vi "Wristband main - Pinch Leap based2.vi"() -> ()   [LabVIEW 2014]
uses:
  Typedef/sensor_data.ctl
  Typedef/flexext_data.ctl
  Typedef/pinch_data.ctl
  SubVIs/Save Blocks - 2D.vi
  <vilib>/MakerHub/LINX/Public/Peripherals/Analog/Analog Read N Chans.vi
  <vilib>/MakerHub/LINX/LMH-LINX.lvlib
panel:
  out "Pinch cluster":T1
  in  "X Scale.Range:Maximum":dbl=200.0 format="%#_13g"
  in  "X Scale.Range:Minimum":dbl format="%#_13g"
  in  "X-scale change":bool
  in  "Clear Plot":bool
  in  "Acquire":bool
  in  "Tacq":u32=50 caption="Acquisition Interval" min=50 max=10000 step=50 format="%.0fms"
  in  "N pts":i32=500
  in  "Session name":string="Sessione Mat"
  in  "Save to path":path=path "C:/Users/Arquilla/Documents/Matteo/Documents/Matteo/Università/Campus Biomedico/Tesi Magistrale/smart wrist save"
  out "Leap \nConnected?":bool=TRUE caption="Leap Motion"
  in  "Arduino Port":refnum<visa-resource-name>
  out "Status":bool caption="Arduino"
  out "Sensor Chart":T2(graph)
  out "Grab Strength":u8
  out "Flexext cluster":T3
  out "Sensor Data":T4={"Sensor  Chan 0"=1.66015625, "Sensor Chan 1"=2.060546875, "Sensor Chan 2"=2.099609375, "Sensor Chan 3"=2.12890625, "Sensor Chan 4"=2.0751953125, "Sensor Chan 5"=1.8115234375}
  in  "Exit":bool
  out "Event Chart":T5(graph)
  # "Connection panel"
  # "Acquisition panel"
  # "Save settings"
  # "Connection status"
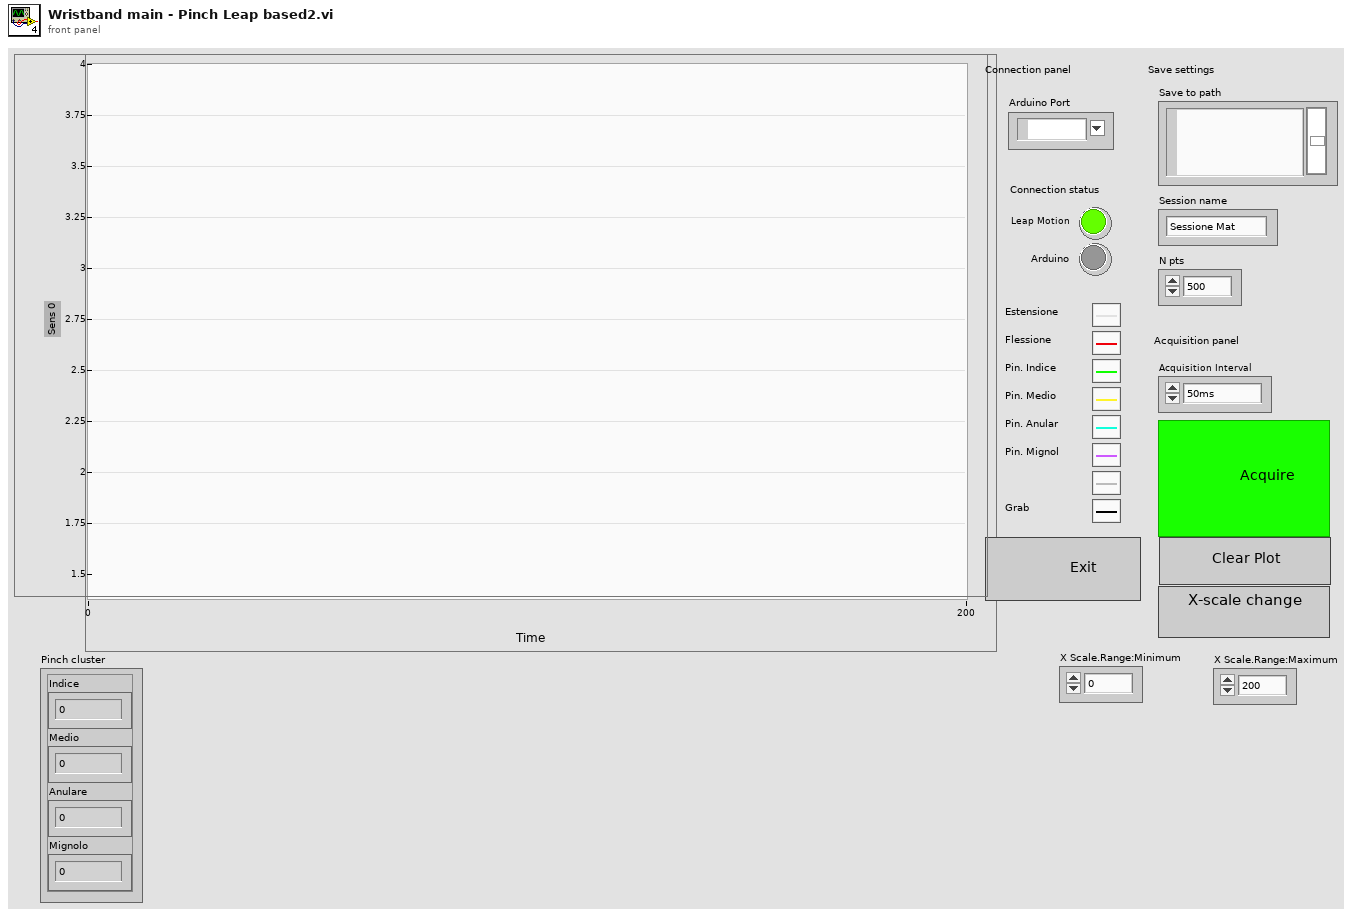
[diagram p1: front panel]
types:
  T1 = typedef "pinch_data.ctl" = cluster{"Indice":u8, "Medio":u8, "Anulare":u8, "Mignolo":u8}
  T2 = cluster{"Sensor  Chan 0":dbl, "Sensor Chan 2":dbl, "Sensor Chan 4":dbl, "Sensor Chan 5":dbl}
  T3 = typedef "flexext_data.ctl" = cluster{"Estensione":u8, "Flessione":u8}
  T4 = typedef "Sensor_data.ctl" = cluster{"Sensor  Chan 0":dbl, "Sensor Chan 1":dbl, "Sensor Chan 2":dbl, "Sensor Chan 3":dbl, "Sensor Chan 4":dbl, "Sensor Chan 5":dbl}
  T5 = cluster{"Estensione":u8, "Flessione":u8, "Indice":u8, "Medio":u8, "Anulare":u8, "Mignolo":u8, "Grab Strength":u8}
  T6 = typedef "LMH-LINX.lvlib/LINX Ref.ctl" = cluster{"Platform":T7, "Interface":T8, "LINX Device Config":T9}
  T7 = typedef "LMH-LINX.lvlib/Platform.ctl" = enum16{"LINX", "myRIO"}
  T8 = typedef "LMH-LINX.lvlib/Interface.ctl" = enum16{"Serial", "TCP"}
  T9 = typedef "LMH-LINX.lvlib/Device.lvlib/LINX Device Config.ctl" = cluster{"Interface":T8, "COM Port":refnum<visa-resource-name>, "TCP Configuration":T10, "Device Family":u8, "Device ID":u8, "Device Name":string, "TCP Ref":refnum<k5>, "Channels":T11}
  T10 = typedef "LMH-LINX.lvlib/Device.lvlib/TCP Config.ctl" = cluster{"IP Address":string, "Port":u16}
  T11 = typedef "LMH-LINX.lvlib/Channels.ctl" = cluster{"DI":u8[], "DO":u8[], "AI":u8[], "AO":u8[], "PWM":u8[], "QE":u8[], "UART":u8[], "I2C 2":u8[], "SPI":u8[], "CAN":u8[], "Servo":u8[], "AI Ref (V)":dbl, "AO Ref (V)":dbl, "AO Resolution (Bits)":u8}
  T12 = typedef "Leap Handle.ctl" = cluster{"LeapCSharp":refnum<k24>}
  T13 = cluster{"Estensione":u8, "Flessione":u8, "Indice":u8, "Medio":u8, "Anulare":u8, "Mignolo":u8, "Grab Strength":u8}[]
  T14 = cluster{"Sensor  Chan 0":dbl, "Sensor Chan 2":dbl, "Sensor Chan 4":dbl, "Sensor Chan 5":dbl}[]
  T15 = cluster{"Sensor  Chan 0":dbl, "Sensor Chan 1":dbl, "Sensor Chan 2":dbl, "Sensor Chan 3":dbl}
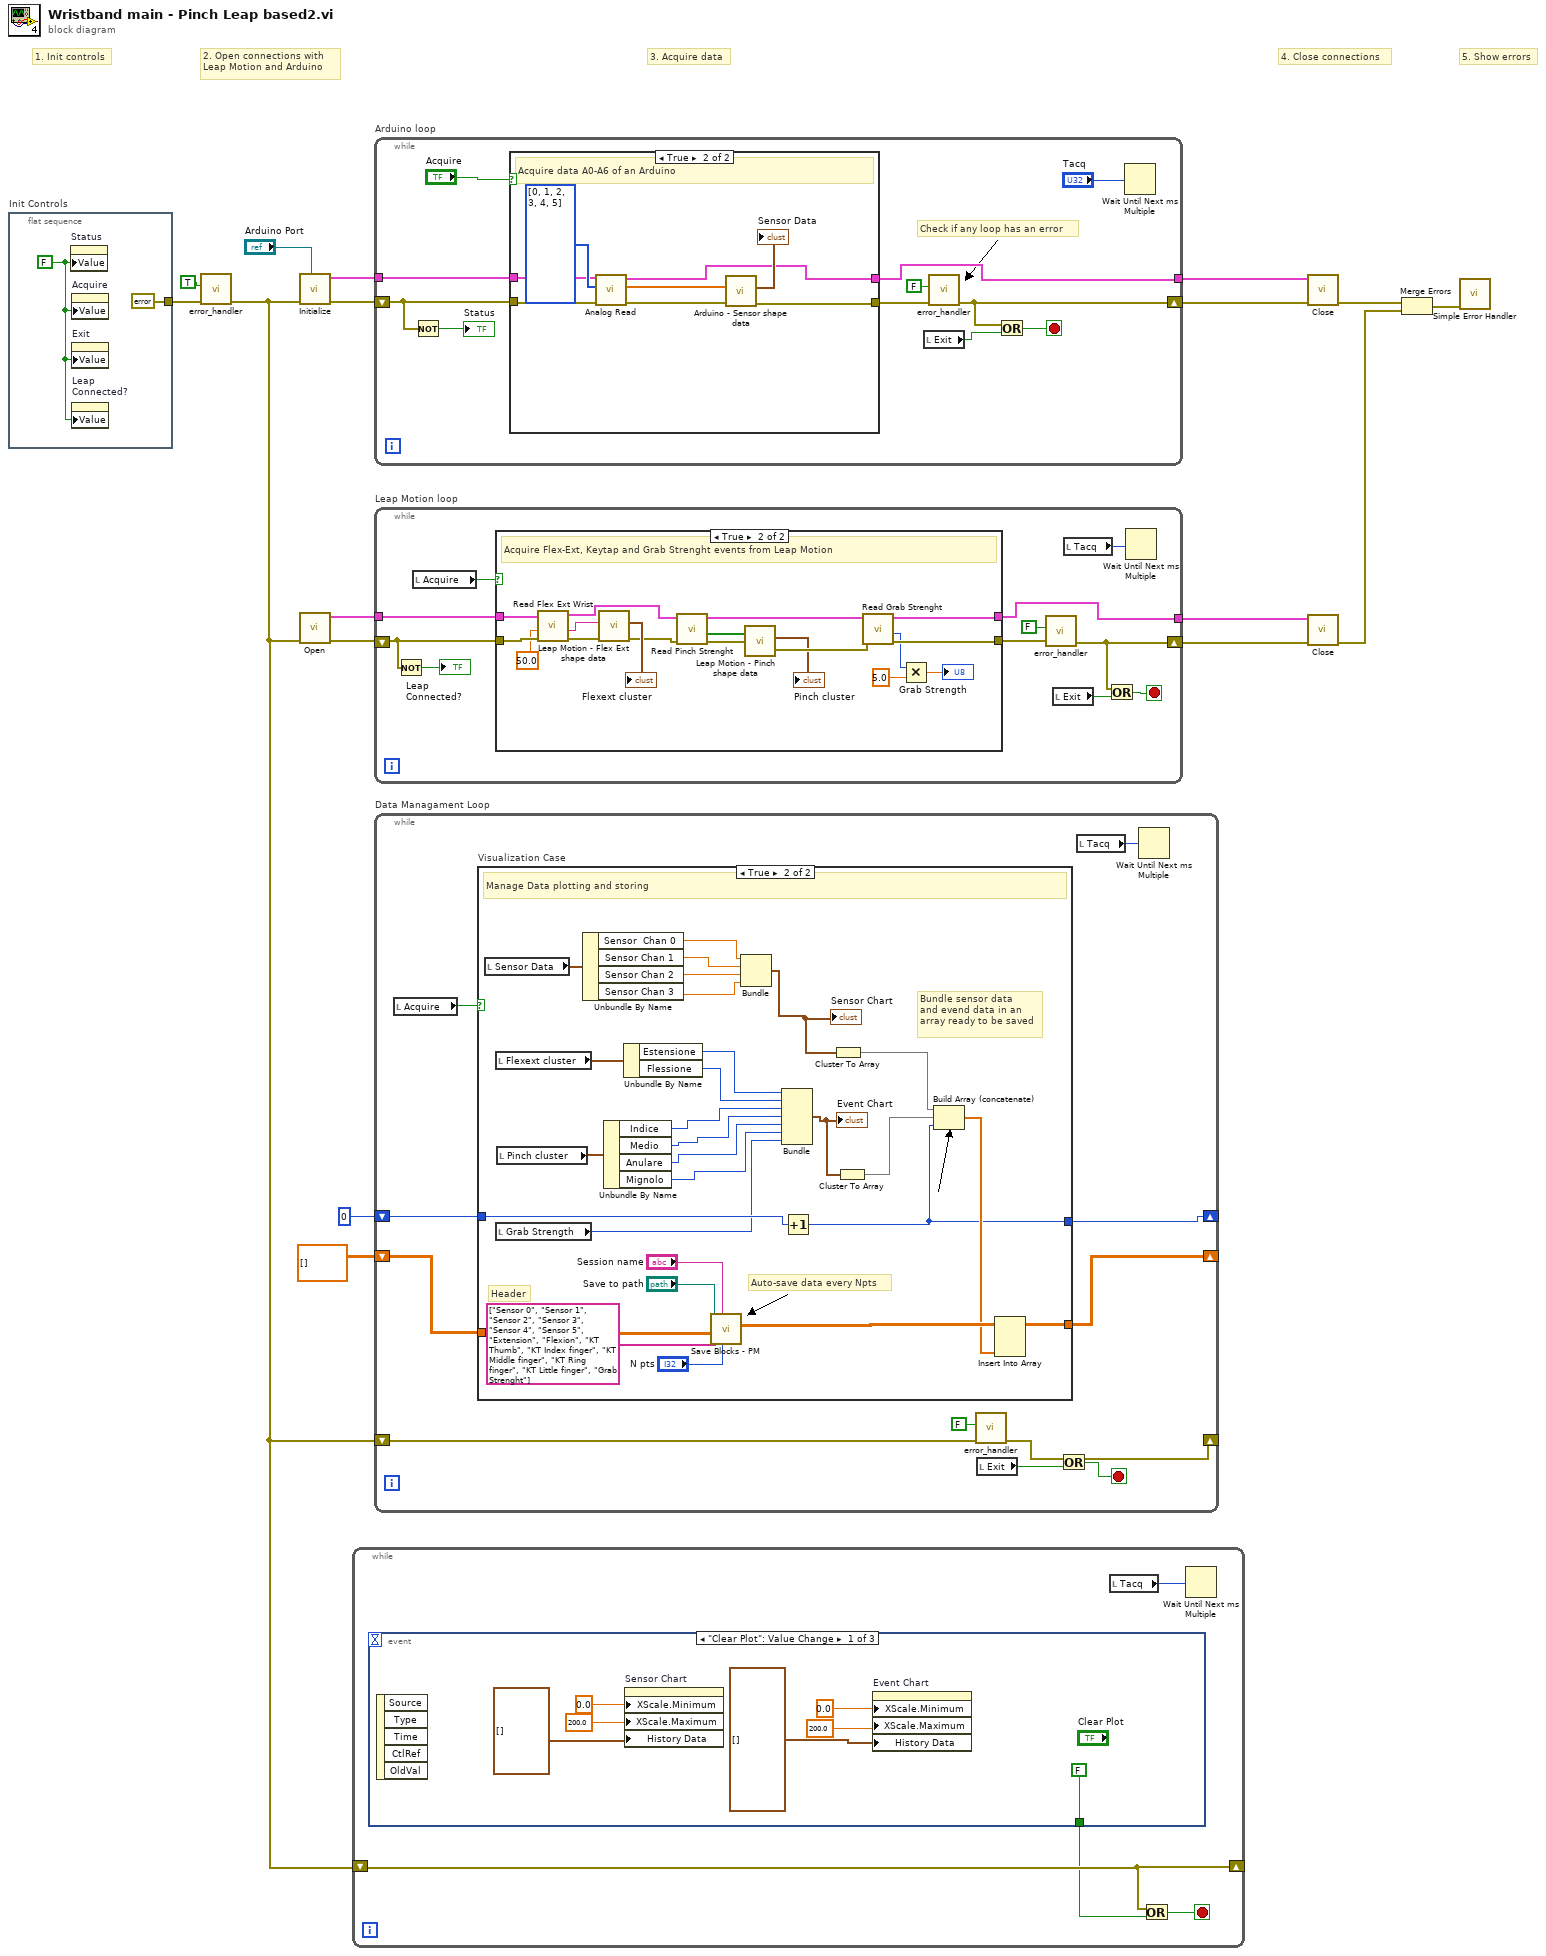
[diagram p0: block diagram]
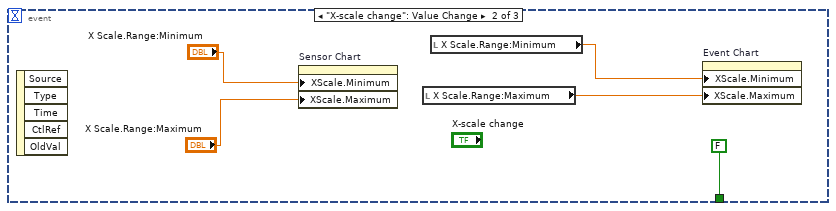
[diagram p2: hidden frame]
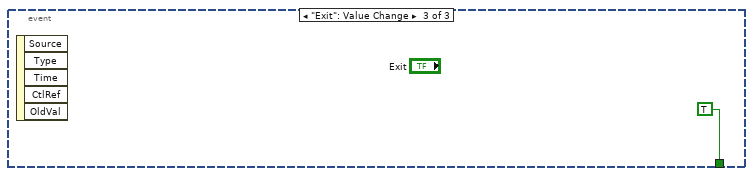
[diagram p3: hidden frame]
diagram:
  # "5. Show errors"
  # "4. Close connections"
  # "3. Acquire data"
  # "2. Open connections with\nLeap Motion and Arduino"
  # "1. Init controls"
  n1 = flat-sequence "Init Controls" {
    tunnel: [errorcluster {"status"=FALSE, "code"=0, "source"=""} ("Error In")] -> w8
    frame #0 {
      w18 = FALSE ("Status")
      n2 = property on="Status" class="Bool (strict)"("Value"=w18) -> ()  [unwired: 2 in, 2 out]
      n3 = property on="Acquire" class="Bool (strict)"("Value"=w18) -> ()  [unwired: 2 in, 2 out]
      n4 = property on="Exit" class="Bool (strict)"("Value"=w18) -> ()  [unwired: 2 in, 2 out]
      n5 = property on="Leap \nConnected?" class="Bool (strict)"("Value"=w18) -> ()  [unwired: 2 in, 2 out]
    }
  }
  n6 = call "error_handler.vi"("Error In"=w8, "Reset"=TRUE) -> ("Error Out"=w2:errorcluster)  [unwired: 9 in]
  n7 = call <vilib>:"Initialize.vi"("Serial Port"="Arduino Port", "Error In"=w2) -> ("Error Out"=w16:errorcluster, "LINX Ref"=w17:T6)  [unwired: 7 in, 1 out]
  n8 = call "Open.vi"("Error In"=w2) -> ("Error Out"=w11:errorcluster, "Leap Handle"=w12:T12)  [unwired: 9 in]
  n9 = while {
    shift-right: [w21] -> _
    shift-left: w2 -> [w21]
    stop <- w22 stop-if-true
    n10 = event shown="[0] \"Clear Plot\": Value Change" {
      selector: _ -> [_ _ _]
      dyn-events: _ -> [_ _ _]
      timeout: _ -> [_ _ _]
      tunnel: [FALSE FALSE TRUE] -> w20
      event "Clear Plot": Value Change {
        n11 = event-data() -> ()  [unwired: 1 in, 5 out]
        n12 = property on="Sensor Chart" class="WFChart (strict)"("XScale.Minimum"=0.0 ("X Scale.Range:Minimum"), "XScale.Maximum"=200.0 ("X Scale.Range:Maximum"), "History Data"=T14 []) -> ()  [unwired: 2 in, 2 out]
        n13 = property on="Event Chart" class="WFChart (strict)"("XScale.Minimum"=0.0 ("X Scale.Range:Minimum"), "XScale.Maximum"=200.0 ("X Scale.Range:Maximum"), "History Data"=T13 []) -> ()  [unwired: 2 in, 2 out]
      }
      event "X-scale change": Value Change {
        n14 = event-data() -> ()  [unwired: 1 in, 5 out]
        n15 = property on="Sensor Chart" class="WFChart (strict)"("XScale.Minimum"="X Scale.Range:Minimum", "XScale.Maximum"="X Scale.Range:Maximum") -> ()  [unwired: 2 in, 2 out]
        n16 = local read "X Scale.Range:Maximum"() -> (w31:dbl)
        n17 = local read "X Scale.Range:Minimum"() -> (w34:dbl)
        n18 = property on="Event Chart" class="WFChart (strict)"("XScale.Minimum"=w34, "XScale.Maximum"=w31) -> ()  [unwired: 2 in, 2 out]
      }
      event "Exit": Value Change {
        n19 = event-data() -> ()  [unwired: 1 in, 5 out]
      }
    }
    n20 = local read "Tacq"() -> (w23:u32)
    n21 = Or(x=w21, y=w20) -> (x .or. y?=w22:bool)
    n22 = Wait Until Next ms Multiple(millisecond multiple=w23) -> ()  [unwired: 1 out]
  }
  n23 = while "Arduino loop" {
    tunnel: w17 -> [w46]
    tunnel: [w39] -> w13
    shift-right: [w40] -> w14
    shift-left: w16 -> [w43]
    stop <- w45 stop-if-true
    # "Check if any loop has an error"
    n24 = Not(x=w43) -> (.not. x?=→"Status":bool)
    n25 = case shown="True" "Acquire" {
      tunnel: w46 -> [w48 w55]
      tunnel: w43 -> [w49 w57]
      tunnel: [w48 w50] -> w39
      tunnel: [w49 w53] -> w41
      frame False {
        # "Idle"
      }
      frame True {
        # "Acquire data A0-A6 of an Arduino"
        n26 = call-poly <vilib>:"Analog Read.vi"("Error In"=w57, "AI Channel(s)"=u8[] [0, 1, 2, 3, 4, 5], "LINX Resource"=w55) -> ("Error Out"=w54:errorcluster, "Voltages"=w52:dbl[], "LINX Resource"=w50:T6)  [unwired: 5 in, 1 out]
        n27 = call "Arduino - Sensor shape data.vi"("Error In"=w54, "Sensor Data in"=w52) -> ("Error Out"=w53:errorcluster, "Sensor Data Out"=→"Sensor Data":T4)  [unwired: 8 in]
      }
    }
    n28 = local read "Exit"() -> (w37:bool)
    n29 = call "error_handler.vi"("Error In"=w41, "Reset"=FALSE) -> ("Error Out"=w40:errorcluster)  [unwired: 9 in]
    n30 = Or(x=w40, y=w37) -> (x .or. y?=w45:bool)
    n31 = Wait Until Next ms Multiple(millisecond multiple="Tacq") -> ()  [unwired: 1 out]
  }
  n32 = while "Leap Motion loop" {
    tunnel: w12 -> [w66]
    tunnel: [w60] -> w10
    shift-right: [w62] -> w9
    shift-left: w11 -> [w59]
    stop <- w67 stop-if-true
    n33 = Not(x=w59) -> (.not. x?=→"Leap \nConnected?":bool)
    n34 = local read "Acquire"() -> (w64:bool)
    n35 = case shown="True" w64 {
      tunnel: w66 -> [w70 w88]
      tunnel: w59 -> [w69 w87]
      tunnel: [w70 w82] -> w60
      tunnel: [w69 w81] -> w63
      frame False {
        # "Idle"
      }
      frame True {
        # "Acquire Flex-Ext, Keytap and Grab Strenght events from Leap Motion"
        n36 = call "Read Flex Ext Wrist.vi"("Error In"=w87, "Flex Extension threshold"=sgl 50.0, "Leap Handle In"=w88) -> ("Error Out"=w85:errorcluster, "Wrist Flextion/Extension"=w84:string, "Leap Handle Out"=w77:T12)  [unwired: 4 in]
        n37 = call "Leap Motion - Flex Ext shape data.vi"("Error In"=w85, "Event In"=w84) -> ("Error Out"=w76:errorcluster, "Flexext cluster"=→"Flexext cluster":T3)  [unwired: 8 in]
        n38 = call "Read Pinch Strenght.vi"("Error In"=w76, "Leap Handle In"=w77) -> ("Error Out"=w74:errorcluster, "Finger pinch"=w73:bool[], "Leap Handle Out"=w75:T12)  [unwired: 6 in, 1 out]
        n39 = call "Leap Motion - Pinch shape data.vi"("Error In"=w74, "Pinch"=w73) -> ("Error Out"=w72:errorcluster, "Pinch cluster"=→"Pinch cluster":T1)  [unwired: 8 in]
        n40 = call "Read Grab Strenght.vi"("Error In"=w72, "Leap Handle In"=w75) -> ("Error Out"=w81:errorcluster, "Numeric Palm State"=w78:i32, "Leap Handle Out"=w82:T12)  [unwired: 5 in, 2 out]
        n41 = Multiply(x=w78, y=sgl 5.0) -> (x*y=→"Grab Strength":sgl)
      }
    }
    n42 = call "error_handler.vi"("Error In"=w63, "Reset"=FALSE) -> ("Error Out"=w62:errorcluster)  [unwired: 9 in]
    n43 = local read "Exit"() -> (w68:bool)
    n44 = local read "Tacq"() -> (w65:u32)
    n45 = Or(x=w62, y=w68) -> (x .or. y?=w67:bool)
    n46 = Wait Until Next ms Multiple(millisecond multiple=w65) -> ()  [unwired: 1 out]
  }
  n47 = while "Data Managament Loop" {
    shift-right: [w94] -> _
    shift-left: w2 -> [w95]
    shift-right: [w93] -> _
    shift-left: dbl[][] [] -> [w92]
    shift-right: [w89] -> _
    shift-left: 0 -> [w90]
    stop <- w96 stop-if-true
    n48 = local read "Acquire"() -> (w99:bool)
    n49 = case "Visualization Case" shown="True" w99 {
      tunnel: [w101 w121] -> w93
      tunnel: w92 -> [w101 w119]
      tunnel: w90 -> [w100 w111]
      tunnel: [w100 w110] -> w89
      frame False {
        # "Idle"
      }
      frame True {
        # "Header"
        # "Auto-save data every Npts"
        # "Bundle sensor data\nand evend data in an\narray ready to be saved"
        # "Manage Data plotting and storing"
        n50 = local read "Sensor Data"() -> (w117:T4)
        n51 = local read "Flexext cluster"() -> (w129:T3)
        n52 = local read "Grab Strength"() -> (w104:u8)
        n53 = local read "Pinch cluster"() -> (w109:T1)
        n54 = Unbundle By Name(w117) -> ("Sensor  Chan 0"=w116:dbl, "Sensor Chan 1"=w115:dbl, "Sensor Chan 2"=w114:dbl, "Sensor Chan 3"=w113:dbl)
        n55 = Unbundle By Name(w109) -> ("Indice"=w108:u8, "Medio"=w107:u8, "Anulare"=w106:u8, "Mignolo"=w105:u8)
        n56 = Unbundle By Name(w129) -> ("Estensione"=w128:u8, "Flessione"=w127:u8)
        n57 = call-poly "Save Blocks - PM.vi"("N pts"="N pts", "Session name"="Session name", "2D Data In"=w119, "Column headers"=string[] ["Sensor 0", "Sensor 1", "Sensor 2", "Sensor 3", "Sensor 4", "Sensor 5", "Extension", "Flexion", "KT Thumb", "KT Index finger", "KT Middle finger", "KT Ring finger", "KT Little finger", "Grab Strenght"], "Save to path"="Save to path") -> ("2D Data Out"=w125:dbl[][])  [unwired: 5 in, 1 out]
        n58 = Bundle("Sensor  Chan 0"=w116, "Sensor Chan 1"=w115, "Sensor Chan 2"=w114, "Sensor Chan 3"=w113) -> (w112:T15)  [unwired: 1 in]
        "Sensor Chart" <- w112
        n59 = Bundle("Estensione"=w128, "Flessione"=w127, "Indice"=w108, "Medio"=w107, "Anulare"=w106, "Mignolo"=w105, "Grab Strength"=w104) -> (w103:T5)  [unwired: 1 in]
        "Event Chart" <- w103
        n60 = Increment(x=w111) -> (x+1=w110:i32)
        n61 = Cluster To Array(cluster=w112) -> (array=w126:dbl[])
        n62 = Cluster To Array(cluster=w103) -> (array=w102:u8[])
        n63 = Build Array (concatenate)(w126, w102, w110) -> (w120:dbl[])
        n64 = Insert Into Array(array=w125, new element=w120) -> (w121:dbl[][])  [unwired: 2 in]
      }
    }
    n65 = call "error_handler.vi"("Error In"=w95, "Reset"=FALSE) -> ("Error Out"=w94:errorcluster)  [unwired: 9 in]
    n66 = local read "Exit"() -> (w97:bool)
    n67 = Or(x=w94, y=w97) -> (x .or. y?=w96:bool)
    n68 = local read "Tacq"() -> (w91:u32)
    n69 = Wait Until Next ms Multiple(millisecond multiple=w91) -> ()  [unwired: 1 out]
  }
  n70 = call <vilib>:"Close.vi"("Error In"=w14, "LINX Resource"=w13) -> ("Error Out"=w5:errorcluster)  [unwired: 8 in, 1 out]
  n71 = call <vilib>:"Close.vi"("Error In"=w9, "Leap Handle"=w10) -> ("Error Out"=w4:errorcluster)  [unwired: 9 in]
  n72 = Merge Errors(w5, w4) -> (w6:errorcluster)
  n73 = call <vilib>:"Simple Error Handler.vi"("error in (no error)"=w6) -> ()  [unwired: 4 in, 5 out]
